vi "ServoCommands.vi"(8 "error in":errorcluster, 9 "milliseconds to wait \nfor servo to change":u32=10, 10 "State":T2(ring), 11 "FPGA VI Reference In":T1) -> (0 "error out":errorcluster)   [LabVIEW 2012]
uses:
  FPGA_ref.ctl
panel:
  in  "milliseconds to wait\nfor flipper/latch":u32=1000
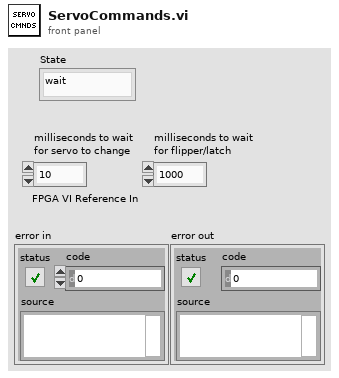
[diagram p1: front panel]
types:
  T1 = typedef "FPGA_ref.ctl" = refnum<k20>
  T2 = enum16{"wait", "open", "close", "lift", "lower", "pickup", "Flip", "UnFlip", "Latch", "UnLatch"}
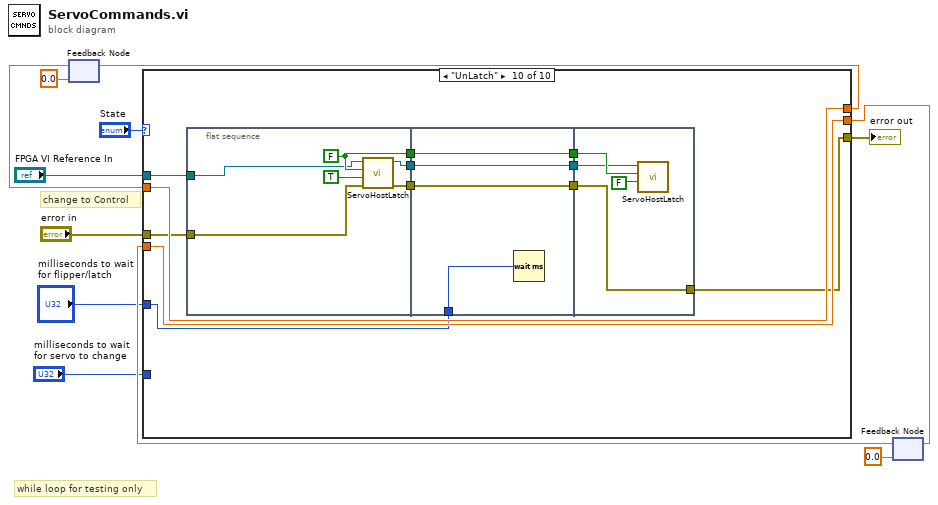
[diagram p0: block diagram]
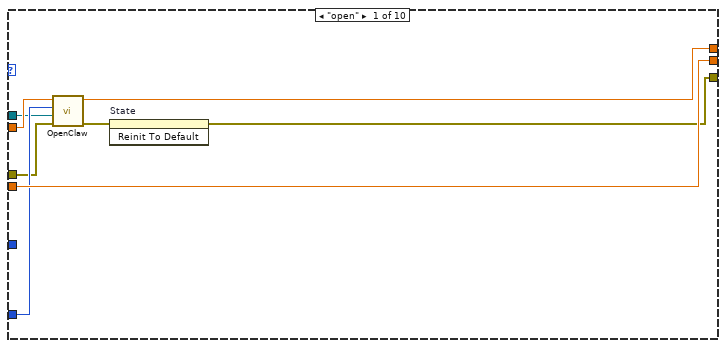
[diagram p2: hidden frame]
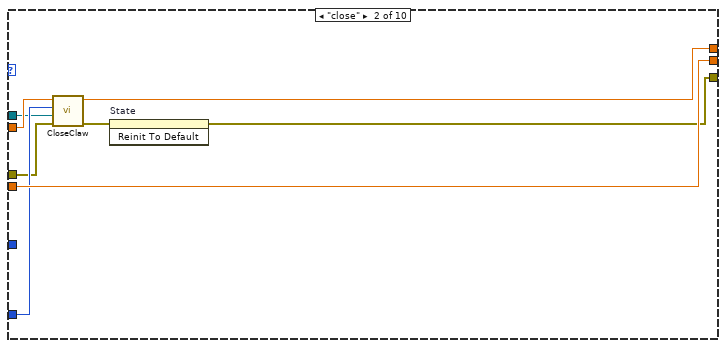
[diagram p3: hidden frame]
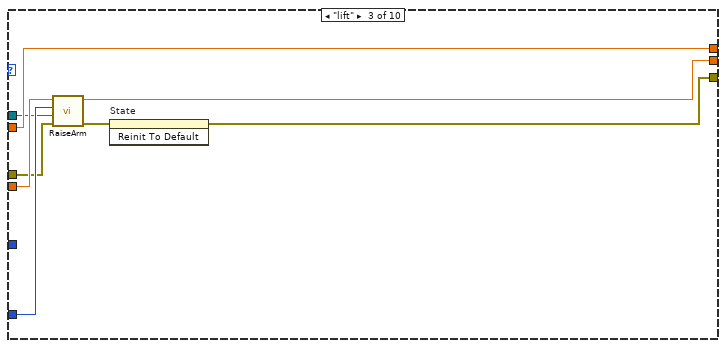
[diagram p4: hidden frame]
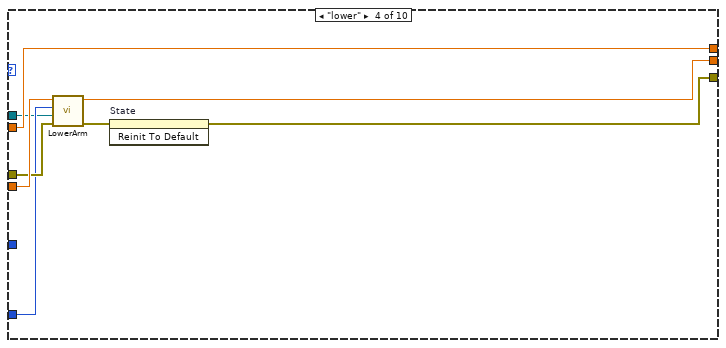
[diagram p5: hidden frame]
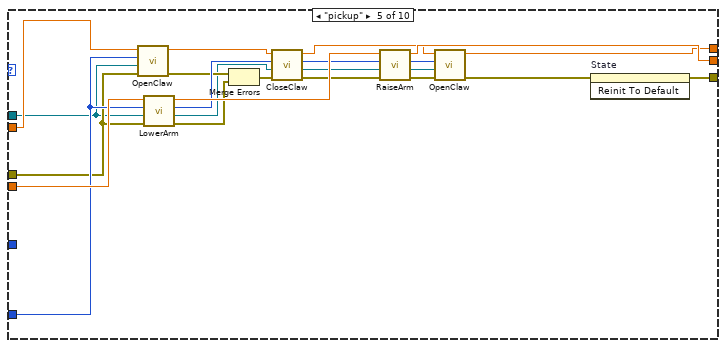
[diagram p6: hidden frame]
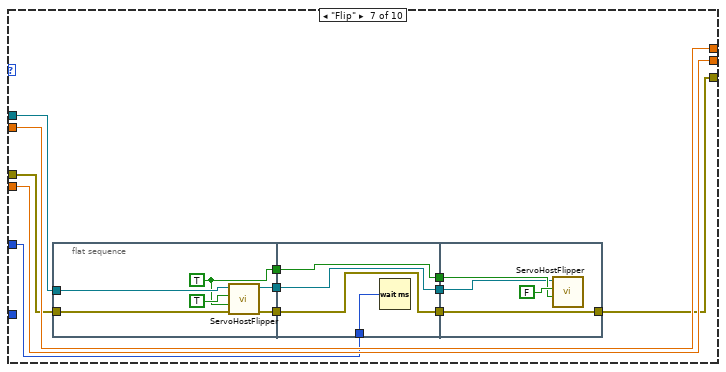
[diagram p8: hidden frame]
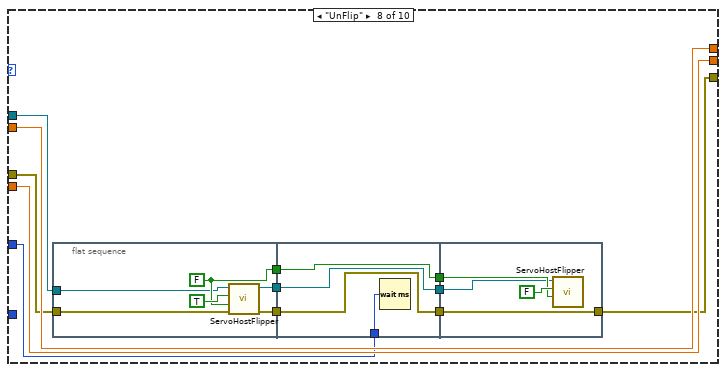
[diagram p9: hidden frame]
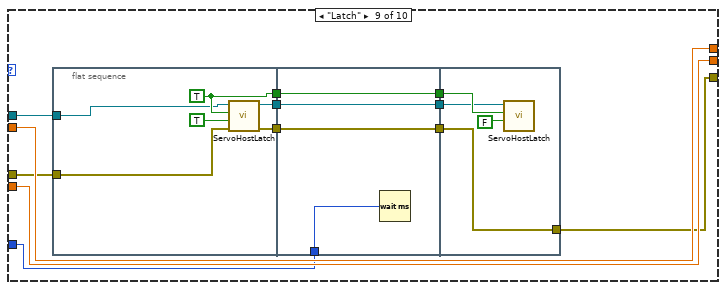
[diagram p10: hidden frame]
diagram:
  # "change to Control"
  # "while loop for testing only"
  n1 = feedback #1(0.0) -> (w8:dbl)
  n2 = feedback #2(0.0) -> (w10:dbl)
  n3 = case shown="\"UnLatch\"" "State" {
    tunnel: "error in" -> [w17 w25 w33 w42 w54 w68 w78 w99 w125 w151]
    tunnel: "milliseconds to wait \nfor servo to change" -> [w19 w27 w34 w40 w55 _ _ _ _ _]
    tunnel: [w20 w28 w32 w41 w65 w69 w82 w107 w133 w159] -> w9
    tunnel: w10 -> [w20 w28 w35 w43 w67 w69 w82 w107 w133 w159]
    tunnel: w8 -> [w18 w26 w36 w44 w53 w70 w81 w108 w134 w160]
    tunnel: [w16 w24 w36 w44 w63 w70 w81 w108 w134 w160] -> w7
    tunnel: [w14 w22 w30 w38 w56 w68 w79 w100 w124 w150] -> w11
    tunnel: "FPGA VI Reference In" -> [w13 w21 w29 w37 w45 _ w80 w98 w126 w152]
    tunnel: "milliseconds to wait\nfor flipper/latch" -> [_ _ _ _ _ _ w71 w97 w123 w149]
    frame "open" {
      n4 = call "OpenClaw.vi"("error in"=w17, "FPGA VI Reference In"=w13, "milliseconds to wait \nfor servo to change"=w19, "Old Angle"=w18) -> ("error out"=w15:errorcluster, "New Angle"=w16:dbl)  [unwired: 4 in, 2 out]
      n5 = invoke on="State" class="Enum (strict)" method="Reinit To Default"(error in=w15) -> (error out=w14:errorcluster)  [unwired: 2 in, 2 out]
    }
    frame "close" {
      n6 = call "CloseClaw.vi"("error in"=w25, "FPGA VI Reference In"=w21, "milliseconds to wait \nfor servo to change"=w27, "Old Angle"=w26) -> ("error out"=w23:errorcluster, "New Angle"=w24:dbl)  [unwired: 4 in, 2 out]
      n7 = invoke on="State" class="Enum (strict)" method="Reinit To Default"(error in=w23) -> (error out=w22:errorcluster)  [unwired: 2 in, 2 out]
    }
    frame "lift" {
      n8 = call "RaiseArm.vi"("error in"=w33, "FPGA VI Reference In"=w29, "milliseconds to wait \nfor servo to change"=w34, "Old Angle"=w35) -> ("error out"=w31:errorcluster, "New Angle"=w32:dbl)  [unwired: 4 in, 2 out]
      n9 = invoke on="State" class="Enum (strict)" method="Reinit To Default"(error in=w31) -> (error out=w30:errorcluster)  [unwired: 2 in, 2 out]
    }
    frame "lower" {
      n10 = call "LowerArm.vi"("error in"=w42, "FPGA VI Reference In"=w37, "milliseconds to wait \nfor servo to change"=w40, "Old Angle"=w43) -> ("error out"=w39:errorcluster, "New Angle"=w41:dbl)  [unwired: 4 in, 2 out]
      n11 = invoke on="State" class="Enum (strict)" method="Reinit To Default"(error in=w39) -> (error out=w38:errorcluster)  [unwired: 2 in, 2 out]
    }
    frame "pickup" {
      n12 = call "OpenClaw.vi"("error in"=w54, "FPGA VI Reference In"=w45, "milliseconds to wait \nfor servo to change"=w55, "Old Angle"=w53) -> ("error out"=w50:errorcluster, "New Angle"=w52:dbl)  [unwired: 4 in, 2 out]
      n13 = call "LowerArm.vi"("error in"=w54, "FPGA VI Reference In"=w45, "milliseconds to wait \nfor servo to change"=w55, "Old Angle"=w67) -> ("error out"=w49:errorcluster, "FPGA VI Reference Out 2"=w48:T1, "milliseconds to wait \nfor servo to change Out"=w60:u32, "New Angle"=w66:dbl)  [unwired: 4 in]
      n14 = Merge Errors(w50, w49) -> (w51:errorcluster)
      n15 = call "CloseClaw.vi"("error in"=w51, "FPGA VI Reference In"=w48, "milliseconds to wait \nfor servo to change"=w60, "Old Angle"=w52) -> ("error out"=w62:errorcluster, "FPGA VI Reference Out"=w47:T1, "milliseconds to wait \nfor servo to change out"=w59:u32, "New Angle"=w64:dbl)  [unwired: 4 in]
      n16 = call "RaiseArm.vi"("error in"=w62, "FPGA VI Reference In"=w47, "milliseconds to wait \nfor servo to change"=w59, "Old Angle"=w66) -> ("error out"=w61:errorcluster, "FPGA VI Reference Out 2"=w46:T1, "milliseconds to wait \nfor servo to change Out"=w58:u32, "New Angle"=w65:dbl)  [unwired: 4 in]
      n17 = call "OpenClaw.vi"("error in"=w61, "FPGA VI Reference In"=w46, "milliseconds to wait \nfor servo to change"=w58, "Old Angle"=w64) -> ("error out"=w57:errorcluster, "New Angle"=w63:dbl)  [unwired: 4 in, 2 out]
      n18 = invoke on="State" class="Enum (strict)" method="Reinit To Default"(error in=w57) -> (error out=w56:errorcluster)  [unwired: 2 in, 2 out]
    }
    frame "wait", Default {
    }
    frame "Flip" {
      n19 = flat-sequence {
        tunnel: w80 -> [w88]
        tunnel: w78 -> [w86]
        tunnel: [w87] -> w77
        tunnel: [w84] -> w75
        tunnel: [w83] -> w73
        tunnel: w77 -> [w92]
        tunnel: [w92] -> w76
        tunnel: w75 -> [w91]
        tunnel: [w91] -> w74
        tunnel: w73 -> [w90]
        tunnel: [w90] -> w72
        tunnel: w71 -> [w89]
        tunnel: [w96] -> w79
        tunnel: w76 -> [w96]
        tunnel: w74 -> [w94]
        tunnel: w72 -> [w93]
        frame #0 {
          w84 = TRUE ("Hi/Lo")
          n20 = call "ServoHostFlipper.vi"("error in"=w86, "Enable"=w84, "Hi/Lo"=TRUE ("Enable"), "FPGA VI Reference In"=w88) -> ("error out"=w87:errorcluster, "FPGA VI Reference Out"=w83:T1)  [unwired: 6 in]
        }
        frame #1 {
          n21 = Wait (ms)(milliseconds to wait=w89) -> ()  [unwired: 1 out]
        }
        frame #2 {
          n22 = call "ServoHostFlipper.vi"("Enable"=w94, "Hi/Lo"=FALSE ("Enable"), "FPGA VI Reference In"=w93) -> ()  [unwired: 7 in, 2 out]
        }
      }
    }
    frame "UnFlip" {
      n23 = flat-sequence {
        tunnel: [w114] -> w106
        tunnel: [w112] -> w105
        tunnel: [w111] -> w104
        tunnel: w99 -> [w110]
        tunnel: w98 -> [w109]
        tunnel: w106 -> [w118]
        tunnel: [w118] -> w103
        tunnel: w105 -> [w117]
        tunnel: [w117] -> w102
        tunnel: w104 -> [w116]
        tunnel: [w116] -> w101
        tunnel: w97 -> [w115]
        tunnel: [w122] -> w100
        tunnel: w103 -> [w122]
        tunnel: w102 -> [w120]
        tunnel: w101 -> [w119]
        frame #0 {
          w112 = FALSE ("Hi/Lo")
          n24 = call "ServoHostFlipper.vi"("error in"=w110, "Enable"=w112, "Hi/Lo"=TRUE ("Enable"), "FPGA VI Reference In"=w109) -> ("error out"=w114:errorcluster, "FPGA VI Reference Out"=w111:T1)  [unwired: 6 in]
        }
        frame #1 {
          n25 = Wait (ms)(milliseconds to wait=w115) -> ()  [unwired: 1 out]
        }
        frame #2 {
          n26 = call "ServoHostFlipper.vi"("Enable"=w120, "Hi/Lo"=FALSE ("Enable"), "FPGA VI Reference In"=w119) -> ()  [unwired: 7 in, 2 out]
        }
      }
    }
    frame "Latch" {
      n27 = flat-sequence {
        tunnel: [w140] -> w132
        tunnel: [w138] -> w131
        tunnel: [w137] -> w130
        tunnel: w125 -> [w136]
        tunnel: w126 -> [w135]
        tunnel: w132 -> [w144]
        tunnel: [w144] -> w129
        tunnel: w131 -> [w143]
        tunnel: [w143] -> w128
        tunnel: w130 -> [w142]
        tunnel: [w142] -> w127
        tunnel: w123 -> [w141]
        tunnel: [w148] -> w124
        tunnel: w129 -> [w148]
        tunnel: w128 -> [w146]
        tunnel: w127 -> [w145]
        frame #0 {
          w138 = TRUE ("Hi/Lo")
          n28 = call "ServoHostLatch.vi"("error in"=w136, "Enable"=TRUE, "Hi/Lo"=w138, "FPGA VI Reference In"=w135) -> ("error out"=w140:errorcluster, "FPGA VI Reference Out"=w137:T1)  [unwired: 6 in]
        }
        frame #1 {
          n29 = Wait (ms)(milliseconds to wait=w141) -> ()  [unwired: 1 out]
        }
        frame #2 {
          n30 = call "ServoHostLatch.vi"("Enable"=FALSE, "Hi/Lo"=w146, "FPGA VI Reference In"=w145) -> ()  [unwired: 7 in, 2 out]
        }
      }
    }
    frame "UnLatch" {
      n31 = flat-sequence {
        tunnel: [w166] -> w158
        tunnel: [w164] -> w157
        tunnel: [w163] -> w156
        tunnel: w151 -> [w162]
        tunnel: w152 -> [w161]
        tunnel: w158 -> [w170]
        tunnel: [w170] -> w155
        tunnel: w157 -> [w169]
        tunnel: [w169] -> w154
        tunnel: w156 -> [w168]
        tunnel: [w168] -> w153
        tunnel: w149 -> [w167]
        tunnel: [w174] -> w150
        tunnel: w155 -> [w174]
        tunnel: w154 -> [w172]
        tunnel: w153 -> [w171]
        frame #0 {
          w164 = FALSE ("Hi/Lo")
          n32 = call "ServoHostLatch.vi"("error in"=w162, "Enable"=TRUE, "Hi/Lo"=w164, "FPGA VI Reference In"=w161) -> ("error out"=w166:errorcluster, "FPGA VI Reference Out"=w163:T1)  [unwired: 6 in]
        }
        frame #1 {
          n33 = Wait (ms)(milliseconds to wait=w167) -> ()  [unwired: 1 out]
        }
        frame #2 {
          n34 = call "ServoHostLatch.vi"("Enable"=FALSE, "Hi/Lo"=w172, "FPGA VI Reference In"=w171) -> ()  [unwired: 7 in, 2 out]
        }
      }
    }
  }
  "error out" <- w11
  n35 = feedback-in #1(w7) -> ()
  n36 = feedback-in #2(w9) -> ()
